vi "Write Duration temp.vi"(8 "error in (no error)":errorcluster, 10 "Duration temp":u16[][](array[numeric]), 11 "Filter params in":refnum<class "CV-Filter.lvclass">) -> (0 "error out":errorcluster, 3 "Filter params out":refnum<class "CV-Filter.lvclass">)   [LabVIEW 2013, in "CameraVision.lvlib" / "CV-Filter.lvclass"]
uses:
  CV-Filter.lvclass
  CV-Filter.lvclass/CV-Filter.ctl
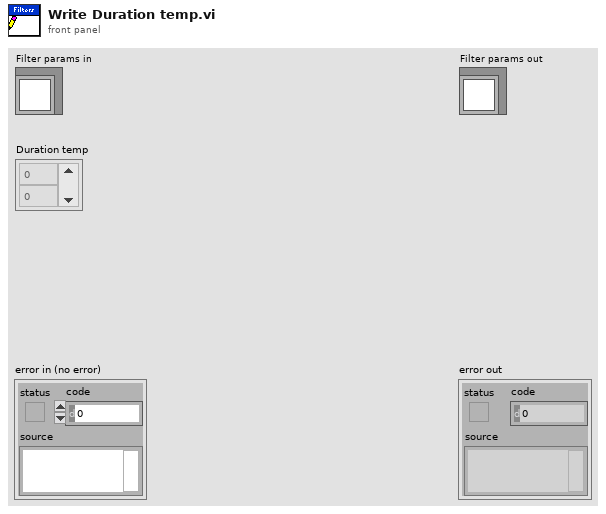
[diagram p1: front panel]
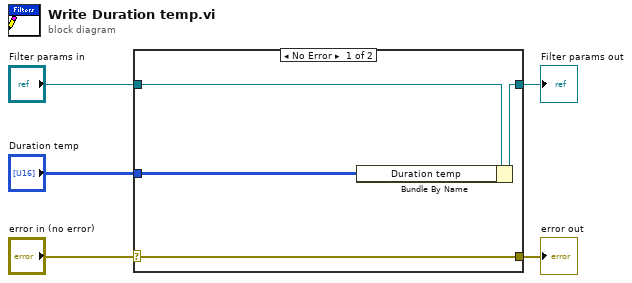
[diagram p0: block diagram]
diagram:
  n1 = case shown="No Error" "error in (no error)" {
    selector: "error in (no error)" -> [w9 w10]
    tunnel: [w9 w10] -> w4
    tunnel: [w7 w11] -> w2
    tunnel: "Filter params in" -> [w8 w11]
    tunnel: "Duration temp" -> [w6 _]
    frame No Error {
      n2 = Bundle By Name(cluster=w8, "Duration temp"=w6) -> (w7:refnum<class "CV-Filter.lvclass">)
    }
    frame Error {
    }
  }
  "error out" <- w4
  "Filter params out" <- w2
